vi "Day11-find_next_flash.vi"(9 "Energy Levels":i32[][](array[numeric]), 11 "Flashed":bool[][](array[boolean])) -> (1 "Flash Location":cluster{i32, i32}, 2 "New Flash?":bool, 3 "Flashed out":bool[][](array[boolean]))   [LabVIEW 2021]
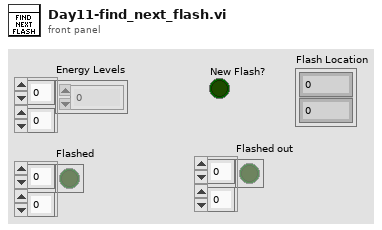
[diagram p1: front panel]
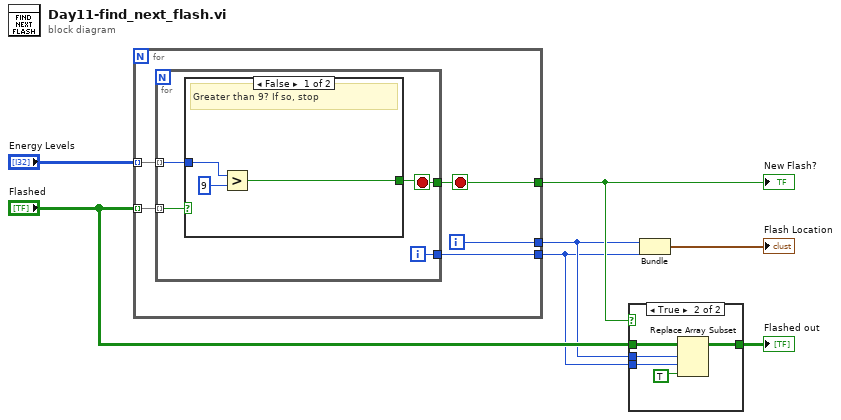
[diagram p0: block diagram]
diagram:
  n1 = for {
    tunnel: "Energy Levels" -> [w12] mode=indexing
    tunnel: "Flashed" -> [w11] mode=indexing
    tunnel: [w10] -> w5
    tunnel: [w9] -> w3
    tunnel: [w8] -> w2
    i -> [w9]
    stop <- w10 stop-if-true
    n2 = for {
      tunnel: w12 -> [w15] mode=indexing
      tunnel: w11 -> [w16] mode=indexing
      tunnel: [w14] -> w8
      tunnel: [w13] -> w10
      i -> [w14]
      stop <- w13 stop-if-true
      n3 = case shown="False" w16 {
        tunnel: w15 -> [w18 _]
        tunnel: [w17 _] -> w13
        frame False {
          # "Greater than 9? If so, stop"
          n4 = Greater?(x=w18, y=9) -> (0:w17:bool)
        }
        frame True {
          # "Already flashed, ignore"
        }
      }
    }
  }
  "New Flash?" <- w5
  n5 = case shown="True" w5 {
    tunnel: "Flashed" -> [w20 w25]
    tunnel: w3 -> [_ w24]
    tunnel: w2 -> [_ w23]
    tunnel: [w20 w21] -> w4
    frame False {
    }
    frame True {
      n6 = Replace Array Subset(array=w25, new element=TRUE, index (row)=w24, index (col)=w23) -> (w21:bool[][])
    }
  }
  "Flashed out" <- w4
  n7 = Bundle(w3, w2) -> (→"Flash Location":cluster{i32, i32})  [unwired: 1 in]
